vi "List Available Packages to Install.vi"(8 "error in":errorcluster, 10 "package name filter":string) -> (0 "error out":errorcluster, 2 "available packages to install":string[][](table))   [LabVIEW 2014, in "NIPM_API.lvlib"]
doc: "Returns a list of all available packages to install.\n\nINPUT(s)\n<B>Package Name Filter</B>: Package name filter: Specifies the glob pattern (e.g. package-abc1, package-abc2, package-abc*, abc) used to filter the returned list of packages. If empty, this VI will return an unfiltered list of packages.\n\nOUTPUT(s)\n<B>Available packages to install</B>: Outputs a list of all available packages to install."
uses:
  NIPM_API.lvlib
panel:
  out "cmd standard output":string
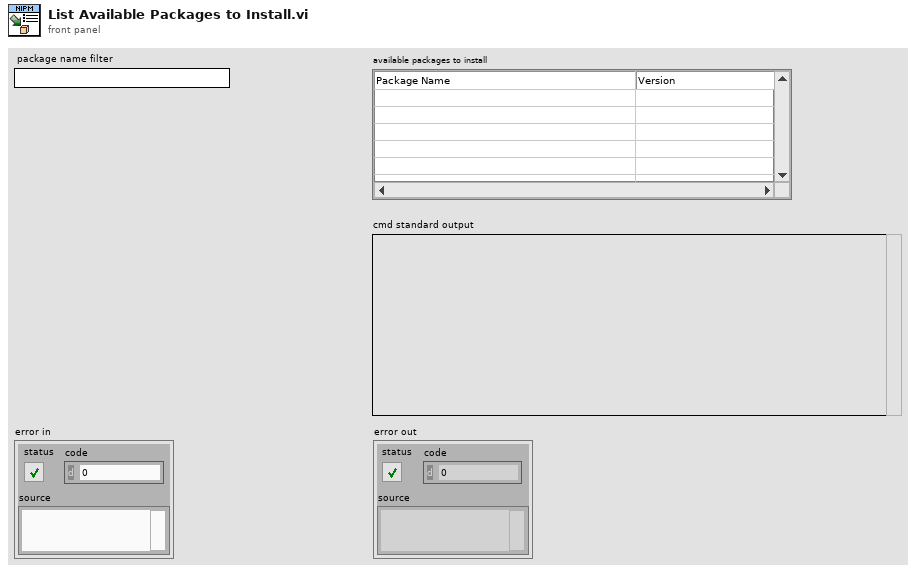
[diagram p1: front panel]
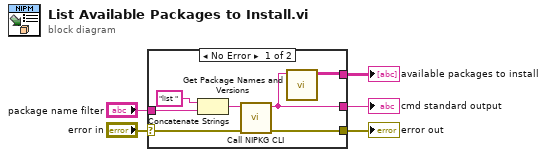
[diagram p0: block diagram]
diagram:
  n1 = case shown="No Error" "error in" {
    selector: "error in" -> [w10 w13]
    tunnel: [w9 _] -> w4
    tunnel: [w12 w13] -> w3
    tunnel: [w8 _] -> w2
    tunnel: "package name filter" -> [w6 _]
    frame No Error {
      n2 = Concatenate Strings("list " ("format string"), w6) -> (w7:string)
      n3 = call "Call NIPKG CLI.vi"("error in (no error)"=w10, "command"=w7) -> ("error out"=w12:errorcluster, "command line standard output"=w9:string)  [unwired: 8 in]
      n4 = call "Get Package Names and Versions.vi"("NIPKG Result"=w9) -> ("Packages"=w8:string[][])  [unwired: 10 in]
    }
    frame Error {
    }
  }
  "error out" <- w3
  "cmd standard output" <- w4
  "available packages to install" <- w2
